vi "idk.vi"() -> ()   [LabVIEW 2020]
doc: "This example shows how to write to addressable LED strip lights.\n\nThis example expects a USB cable connected from your development PC to the Type B USB Jack (next to the power input) on the roboRIO."
uses:
  <vilib>/Rock Robotics/SystemInterfaces/DIO/FPGA_DIOPWMChannel.ctl
panel:
  out "String Length":u16=144
  in  "PWM Channel":T1=enum."PWM 9"
  out "LED Strip":u32[](array[colorbox])
  in  "stop":bool
  # "Set this input before running."
  # "This shows the colors sent."
  # "LED Strip Lights"
  # "This shows wiring for an addressable LED Strip Light. Only one light strip is supported on the roboRIO. Controls WS2812B and compatible strips."
  # "DIN"
  # "+5V"
  # "GND"
  # "^"
  # "^"
  # "^"
  # "^"
  # "LED Strip\nDIN (blue wire)-------\n+5V (red wire)--------\nGND (black wire)-----"
  # "roboRIO\nPWM-9  S \nPWM-9  V\nPWM-9"
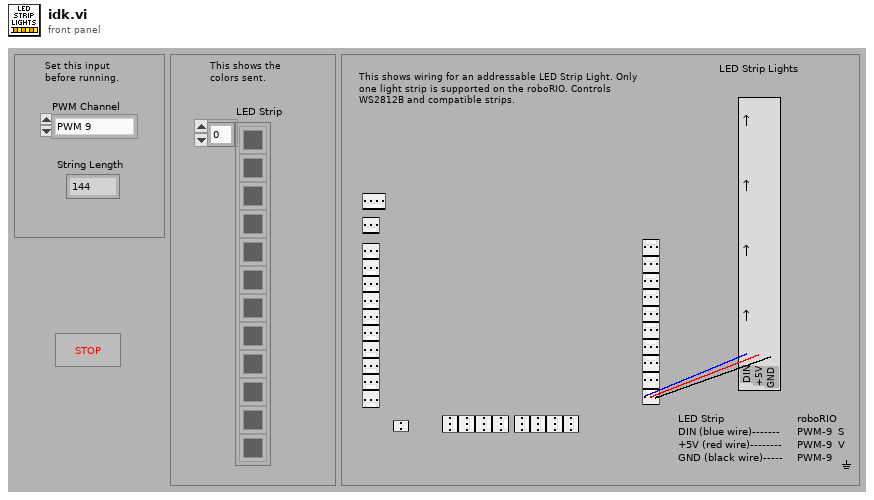
[diagram p1: front panel]
types:
  T1 = typedef "FPGA_DIOPWMChannel.ctl" = enum8{"PWM 0", "PWM 1", "PWM 2", "PWM 3", "PWM 4", "PWM 5", "PWM 6", "PWM 7", "PWM 8", "PWM 9", "PWM MXP 0", "PWM MXP 1", "PWM MXP 2", "PWM MXP 3", "PWM MXP 4", "PWM MXP 5", "PWM MXP 6", "PWM MXP 7", "PWM MXP 8", "PWM MXP 9", "Invalid"}
  T2 = typedef "WPI_PWMDeviceRef.ctl" = cluster{"DeviceStatus":errorcluster, "PWM Channel":T1}
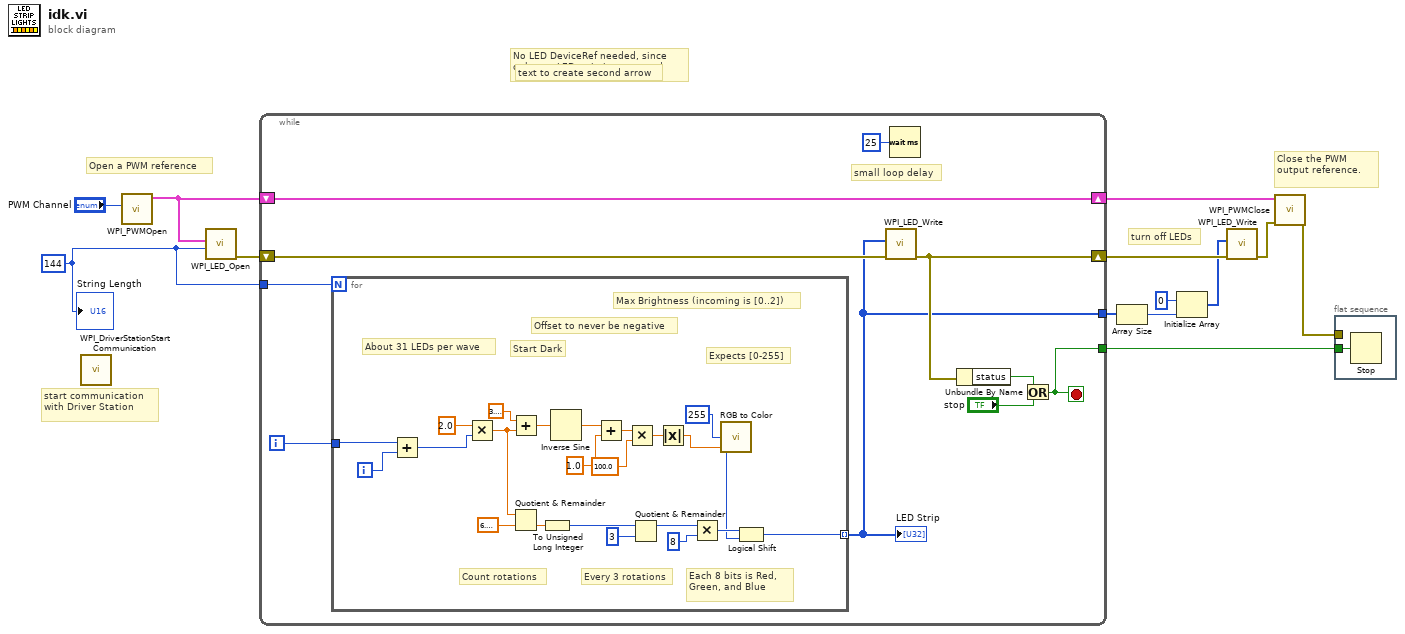
[diagram p0: block diagram]
diagram:
  w1 = u16 144 ("String Length")
  # "turn off LEDs"
  # "No LED DeviceRef needed, since only one LED strip is supported"
  # "Open a PWM reference"
  # "start communication with Driver Station"
  # "Close the PWM output reference."
  # "text to create second arrow"
  n1 = call <vilib>:"WPI_DriverStationStart Communication.vi"() -> ()  [unwired: 3 in, 9 out]
  n2 = call <vilib>:"WPI_PWMOpen.vi"("PWM Channel"="PWM Channel") -> ("PWMDeviceRef"=w10:T2)  [unwired: 9 in, 1 out]
  n3 = call <vilib>:"WPI_LED_Open.vi"("String Length"=w1, "PWMDeviceRef"=w10) -> ("error out"=w11:errorcluster)  [unwired: 9 in]
  n4 = while {
    shift-right: [w19] -> w12
    shift-left: w10 -> [w19]
    tunnel: [w22] -> w13
    shift-right: [w17] -> w8
    shift-left: w11 -> [w18]
    tunnel: w1 -> [w15]
    tunnel: [w14] -> w5
    i -> [w16]
    stop <- w22 stop-if-true
    # "small loop delay"
    n5 = for {
      N: w15 -> [_]
      tunnel: w16 -> [w45]
      tunnel: [w26] -> w14 mode=indexing
      i -> [w46]
      # "Expects [0-255]"
      # "Max Brightness (incoming is [0..2])"
      # "Offset to never be negative"
      # "About 31 LEDs per wave"
      # "Start Dark"
      # "Each 8 bits is Red, Green, and Blue"
      # "Every 3 rotations"
      # "Count rotations"
      n6 = Add(x=w45, y=w46) -> (x+y=w27:i32)
      n7 = Multiply(x=2.0, y=w27) -> (x*y=w44:dbl)
      n8 = Add(x=3.141592653589793, y=w44) -> (x+y=w38:dbl)
      n9 = Quotient & Remainder(x=w44, y=6.283185307179586) -> (floor(x/y)=w40:dbl)  [unwired: 1 out]
      n10 = To Unsigned Long Integer(number=w40) -> (unsigned 32bit integer=w41:u32)
      n11 = Inverse Sine(1:w38) -> (0:w36:dbl)
      n12 = Add(x=w36, y=1.0 ("x")) -> (x+y=w35:dbl)
      n13 = Multiply(x=w35, y=100.0 ("x")) -> (x*y=w37:dbl)
      n14 = Quotient & Remainder(x=w41, y=u32 3) -> (x-y*floor(x/y)=w39:u32)  [unwired: 1 out]
      n15 = Absolute Value(x=w37) -> (abs(x)=w25:dbl)
      n16 = Multiply(x=w39, y=u32 8) -> (x*y=w43:u32)
      n17 = call <vilib>:"RGB to Color.vi"("B"=w25, "G"=u8 255) -> ("Color"=w42:u32)  [unwired: 1 in]
      n18 = Logical Shift(y=w43, x=w42) -> (x << y=w26:u32)
    }
    "LED Strip" <- w14
    n19 = call <vilib>:"WPI_LED_Write.vi"("error in"=w18, "Color Array"=w14) -> ("error out"=w17:errorcluster)  [unwired: 9 in]
    n20 = Wait (ms)(milliseconds to wait=u32 25) -> ()  [unwired: 1 out]
    n21 = Unbundle By Name(w17) -> ("status"=w20:bool)
    n22 = Or(x=w20, y="stop") -> (x .or. y?=w22:bool)
  }
  n23 = Array Size(array=w5) -> (size(s)=w6:i32)
  n24 = Initialize Array(u32 0, w6) -> (w3:u32[])
  n25 = call <vilib>:"WPI_LED_Write.vi"("error in"=w8, "Color Array"=w3) -> ("error out"=w7:errorcluster)  [unwired: 9 in]
  n26 = call <vilib>:"WPI_PWMClose.vi"("error in (no error)"=w7, "PWMDeviceRef"=w12) -> ("error out"=w2:errorcluster)  [unwired: 9 in]
  n27 = flat-sequence {
    tunnel: w13 -> [w47]
    tunnel: w2 -> [_]
    frame #0 {
      n28 = Stop(stop? (T)=w47) -> ()
    }
  }
  "String Length" <- w1
